vi "getAvailableFunctionBlockTypes.vi"(8 "error in (no error)":errorcluster, 11 "IDevice in":refnum<class "IDevice.lvclass">) -> (0 "error out":errorcluster, 2 "Device Types out":T1(c390), 3 "IDevice out":refnum<class "IDevice.lvclass">)   [LabVIEW 2022 SP3, in "openDAQ.lvlib" / "IBaseObject.lvlib" / "IPropertyObject.lvlib" / "IComponent.lvlib" / "IFolder.lvlib" / "IDevice.lvlib" / "IDevice.lvclass"]
uses:
  <instrlib>/openDAQ/Public/Classes/IDevice/IDevice.lvclass
  <instrlib>/openDAQ/Public/Classes/IDevice/IDevice.lvclass/IDevice.ctl
  <instrlib>/openDAQ/Public/Classes/daqCoreTypes/IDict/IDict.lvclass
  <instrlib>/openDAQ/Public/Classes/IFunctionBlockType/IFunctionBlockType.lvclass
  <instrlib>/openDAQ/Binaries/Windows/x86/copendaq32.dll
  <instrlib>/openDAQ/Public/Classes/daqCoreTypes/IDict/Polymorphic/getValueList/getFunctionBlockTypeValueList.vi
  <instrlib>/openDAQ/Public/Classes/daqCoreTypes/IDict/Polymorphic/getKeyList/getStringKeyList.vi
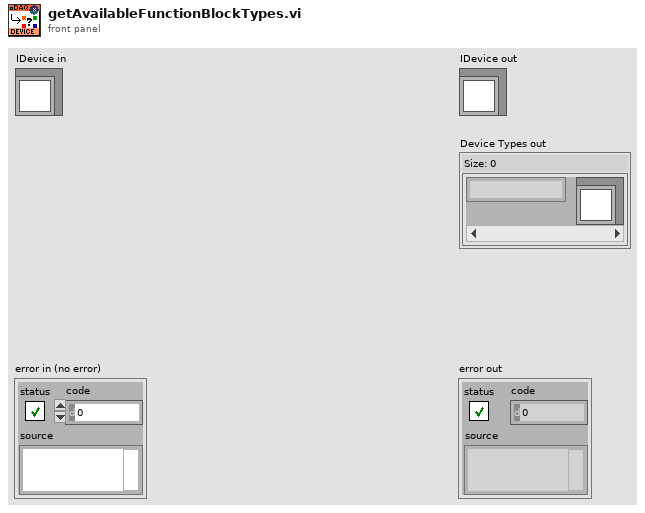
[diagram p1: front panel]
types:
  T1 = map{string, refnum<class "IFunctionBlockType.lvclass">}
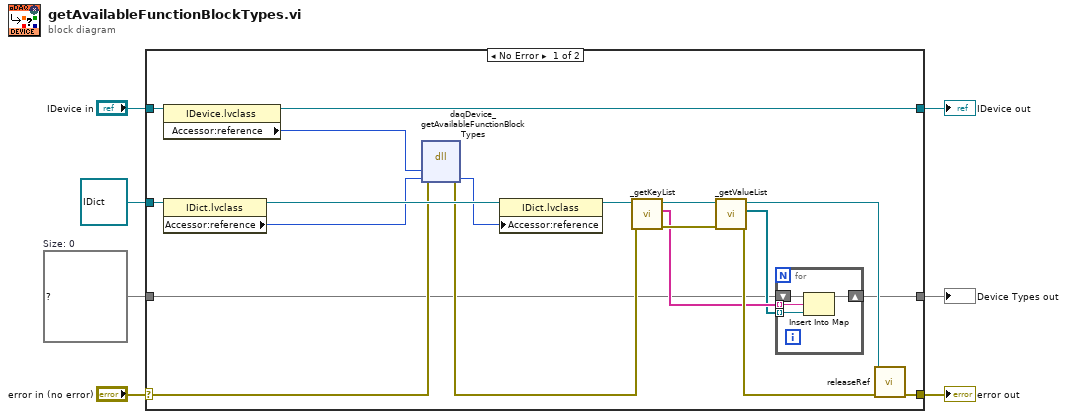
[diagram p0: block diagram]
diagram:
  w2 = T1 {}  # Size: 0
  n1 = case shown="No Error" "error in (no error)" {
    selector: "error in (no error)" -> [w22 w33]
    tunnel: [w13 w33] -> w6
    tunnel: [w21 w32] -> w4
    tunnel: "IDevice in" -> [w24 w32]
    tunnel: refnum<class "IDict.lvclass"> refnum ("openDAQ.lvlib:daqCoreTypes.lvlib:IDict.lvclass") -> [w20 _]
    tunnel: w2 -> [w9 w31]
    tunnel: [w8 w31] -> w1
    frame No Error {
      n2 = property class="IDevice.lvclass"(reference=w24) -> (reference out=w21:refnum<class "IDevice.lvclass">, "Accessor:reference"=w23:i64)  [unwired: 1 in, 1 out]
      n3 = property class="IDict.lvclass"(reference=w20) -> (reference out=w26:refnum<class "IDict.lvclass">, "Accessor:reference"=w19:i64)  [unwired: 1 in, 1 out]
      n4 = dll-call lib="C:/Program Files (x86)/National Instruments/LabVIEW 2022/instr.lib/openDAQ/Binaries/Windows/x86/copendaq*.*" fn="daqDevice_getAvailableFunctionBlockTypes"(error in=w22, "device"=w23, "functionBlockTypes"=w19) -> (error out=w15:errorcluster, "functionBlockTypes"=w25:i64)  [unwired: 4 in, 1 out]
      n5 = property class="IDict.lvclass"(reference=w26, "Accessor:reference"=w25) -> (reference out=w18:refnum<class "IDict.lvclass">)  [unwired: 1 in, 1 out]
      n6 = call-poly <instrlib>:"_getKeyList.vi"("error in (no error)"=w15, "IDict in"=w18) -> ("error out"=w16:errorcluster, "Key List out"=w11:string[], "IDict out"=w17:refnum<class "IDict.lvclass">)  [unwired: 7 in]
      n7 = call-poly <instrlib>:"_getValueList.vi"("error in (no error)"=w16, "IDict in"=w17) -> ("error out"=w14:errorcluster, "Function Block Types out"=w10:refnum<class "IFunctionBlockType.lvclass">[], "IDict out"=w12:refnum<class "IDict.lvclass">)  [unwired: 7 in]
      n8 = for {
        shift-right: [w27] -> w8
        shift-left: w9 -> [w30]
        tunnel: w11 -> [w29] mode=indexing
        tunnel: w10 -> [w28] mode=indexing
        n9 = Insert Into Map(map in=w30, key=w29, value=w28) -> (map out=w27:T1)  [unwired: 2 out]
      }
      n10 = call-dynamic "releaseRef.vi"("error in (no error)"=w14, "IBaseObject in"=w12) -> ("error out"=w13:errorcluster)  [unwired: 9 in]
    }
    frame Error {
    }
  }
  "error out" <- w6
  "IDevice out" <- w4
  "Device Types out" <- w1
